vi "AddEdge.vi"(4 "sink":i32, 5 "source":i32, 9 "VI_AST in":refnum<class "VI_AST.lvclass">) -> (3 "VI_AST out":refnum<class "VI_AST.lvclass">)   [LabVIEW 2014, in "VI_AST.lvclass"]
uses:
  VI_AST.lvclass
  VI_AST.lvclass/VI_AST.ctl
  DAG/DAG/DAG.lvclass
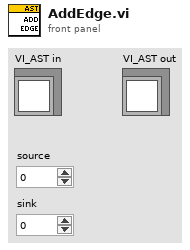
[diagram p1: front panel]
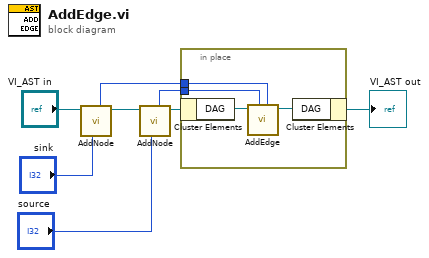
[diagram p0: block diagram]
diagram:
  n1 = call "AddNode.vi"("UID"="sink", "VI_AST in"="VI_AST in") -> ("VI_AST out"=w6:refnum<class "VI_AST.lvclass">, "index"=w3:i32)  [unwired: 6 in]
  n2 = call "AddNode.vi"("UID"="source", "VI_AST in"=w6) -> ("VI_AST out"=w5:refnum<class "VI_AST.lvclass">, "index"=w4:i32)  [unwired: 6 in]
  n3 = in-place {
    in-place-border: w4 -> [w10]
    in-place-border: w3 -> [w9]
    n4 = in-place-cluster #1(w5) -> ("DAG"=w12:refnum<class "DAG.lvclass">)
    n5 = call "AddEdge.vi"("end"=w9, "start"=w10, "DAG in"=w12) -> ("DAG out"=w11:refnum<class "DAG.lvclass">)  [unwired: 6 in]
    n6 = in-place-cluster #1("DAG"=w11) -> (→"VI_AST out":refnum<class "VI_AST.lvclass">)
  }
